vi "DMM Measurement.vi"() -> ()   [LabVIEW 2021]
doc: "This example acquires a single measurement from a National Instruments DMM. Select the measurement function and range. Specify the resolution in digits of precision. The measured value will be displayed in the Measurement indicator. The Boolean indicator will indicate if the measured value is out of range."
uses:
  <instrlib>/niDMM/nidmm.llb/niDMM Configure Measurement Digits.vi
  <instrlib>/niScope/Acquire/niScope Multi Read Cluster.vi
  <instrlib>/niDMM/nidmm.llb/niDMM Function.ctl
  <instrlib>/niDMM/nidmm.llb/niDMM Resolution in Digits.ctl
panel:
  in  "Channel(s)":string="0"
  in  "Scope":refnum<k15>="Dev1" caption="Resource Name(s)"
  out "Waveform Graph":T1(graph)
  out "error out":errorcluster
  in  "error in":errorcluster caption="error in (no error)"
  in  "Resolution in Digits":T2=5.5 items=["3 1/2"=3.5, "4 1/2"=4.5, "5 1/2"=5.5, "6 1/2"=6.5, "7 1/2"=7.5]
  out "Absolute Resolution":dbl format="%#_3p"
  in  "Measurement Type":T3
  out "Signal Out of Range":bool
  in  "Range":dbl=10.0 format="%.2f"
  in  "Device Name":refnum<k15>="Dev1"
  out "Measurement":dbl format="%.6p"
  # "For instructions select File >> VI Properties >> Documentation"
  # "Configuration"
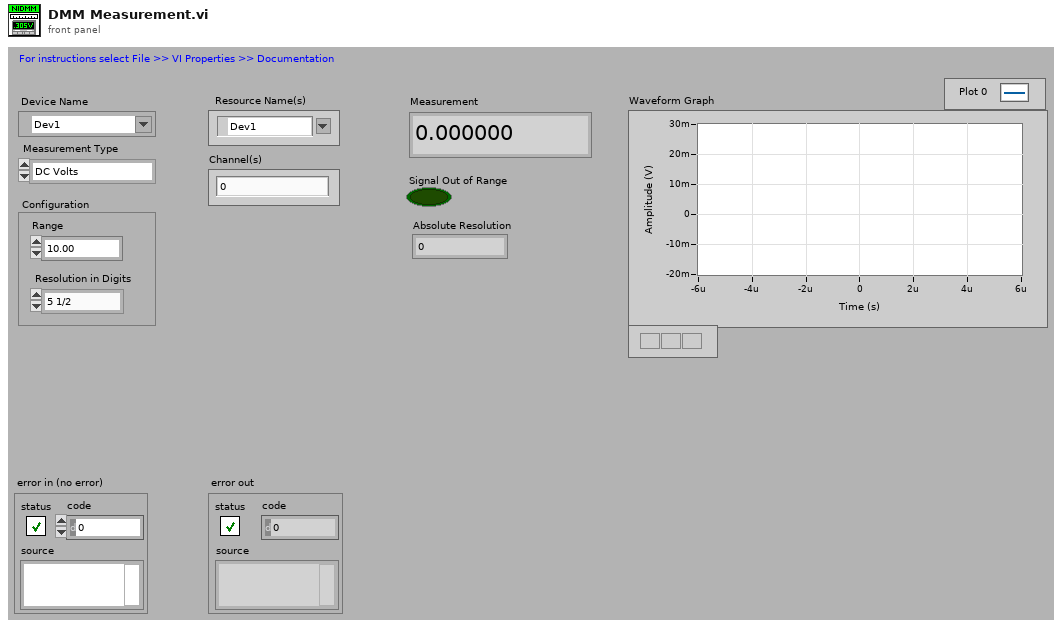
[diagram p1: front panel]
types:
  T1 = cluster{"relativeInitialX":dbl, "xIncrement":dbl, "wfm":dbl[]}[]
  T2 = typedef "niDMM Resolution in Digits.ctl" = dbl
  T3 = typedef "niDMM Function.ctl" = enum16{"DC Volts", "AC Volts", "DC Current", "AC Current", "2-wire Resistance", "4-wire Resistance", "Diode", "Frequency", "Period", "AC Volts DC Coupled", "Capacitance", "Inductance", "Temperature"}
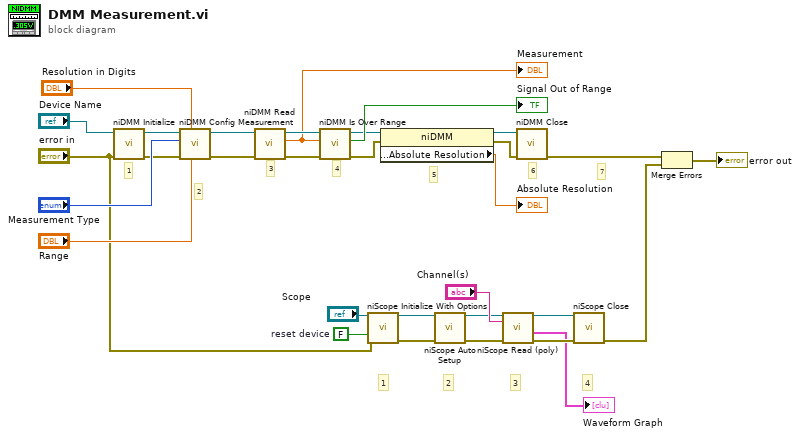
[diagram p0: block diagram]
diagram:
  w7 = FALSE  # reset device
  # "4"
  # "3"
  # "2"
  # "1"
  # "2"
  # "1"
  # "7"
  # "6"
  # "5"
  # "4"
  # "3"
  n1 = call <instrlib>:"niDMM Initialize.vi"("error in (no error)"="error in", "Instrument Descriptor"="Device Name") -> ("error out"=w22:errorcluster, "instrument handle out"=w21:refnum<k15>)  [unwired: 8 in]
  n2 = call-poly <instrlib>:"niDMM Config Measurement.vi"("Range"="Range", "Resolution in Digits"="Resolution in Digits", "error in (no error)"=w22, "Function"="Measurement Type", "instrument handle"=w21) -> ("error out"=w29:errorcluster, "instrument handle out"=w28:refnum<k15>)  [unwired: 5 in]
  n3 = call <instrlib>:"niDMM Read.vi"("error in (no error)"=w29, "instrument handle"=w28) -> ("error out"=w26:errorcluster, "Measurement"=w24:dbl, "instrument handle out"=w27:refnum<k15>)  [unwired: 7 in]
  "Measurement" <- w24
  n4 = call <instrlib>:"niDMM Is Over Range.vi"("error in (no error)"=w26, "Measurement"=w24, "instrument handle"=w27) -> ("error out"=w18:errorcluster, "Over Range?"=→"Signal Out of Range":bool, "instrument handle out"=w20:refnum<k15>)  [unwired: 6 in]
  n5 = call <instrlib>:"niScope Initialize With Options.vi"("resource name"="Scope", "reset device"=w7, "error in"="error in") -> ("instrument handle"=w4:refnum<k15>, "error out"=w5:errorcluster)  [unwired: 11 in]
  n6 = property class="niDMM"(reference=w20, error in=w18) -> (reference out=w19:refnum<k15>, error out=w17:errorcluster, "Configuration:Absolute Resolution"=→"Absolute Resolution":dbl)
  n7 = call <instrlib>:"niScope Auto Setup.vi"("instrument handle"=w4, "error in"=w5) -> ("instrument handle out"=w8:refnum<k15>, "error out"=w9:errorcluster)  [unwired: 12 in]
  n8 = call-poly <instrlib>:"niScope Read (poly).vi"("error in"=w9, "channels"="Channel(s)", "instrument handle"=w8) -> ("error out"=w12:errorcluster, "waveform"=→"Waveform Graph":T1, "instrument handle out"=w13:refnum<k15>)  [unwired: 5 in, 1 out]
  n9 = call <instrlib>:"niDMM Close.vi"("error in (no error)"=w17, "instrument handle"=w19) -> ("error out"=w14:errorcluster)  [unwired: 9 in]
  n10 = call <instrlib>:"niScope Close.vi"("instrument handle"=w13, "error in"=w12) -> ("error out"=w2:errorcluster)  [unwired: 13 in]
  n11 = Merge Errors(w14, w2) -> (→"error out":errorcluster)
